vi "rs3 Set_calibration_table.vi"(8 "error in (no error)":errorcluster, 9 "calibration_Size":i32, 10 "PointerToNewCalibrationTable":u64, 11 "Device in":u64) -> (0 "error out":errorcluster, 1 "error":u64, 3 "Device out":u64)   [LabVIEW 2017, in "libRealSense3.lvlib"]
doc: "STARTS the streaming of a specific sensor, based on the input QUEUE."
uses:
  libRealSense3.lvlib
  realsense2.dll
panel:
  # "RS Set Calibration Table"
  # "(C) 2019 Intel Corp.,  AGJ"
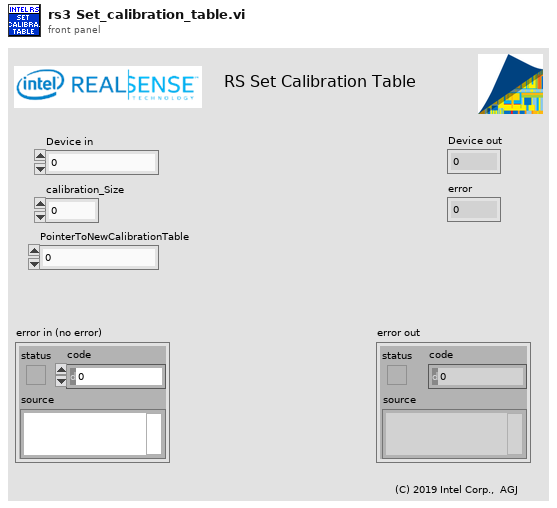
[diagram p1: front panel]
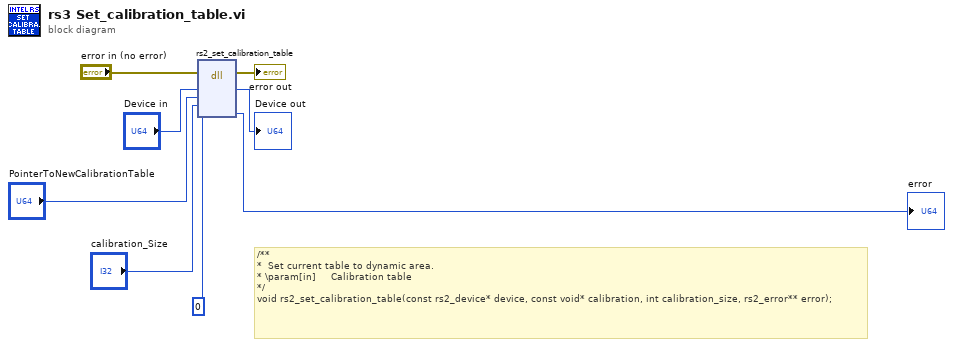
[diagram p0: block diagram]
diagram:
  # "/**\n*  Set current table to dynamic area.\n* \\param[in]     Calibration table\n*/\nvoid rs2_set_calibration_table(const rs2_device* device, const void* calibration, int calibration_size, rs2_error** error);"
  n1 = dll-call lib="C:/Users/agrunnet/Documents/libRealSense6/realsense2.dll" fn="rs2_set_calibration_table"(error in="error in (no error)", "device"="Device in", "CalibrationTable"="PointerToNewCalibrationTable", "calibration_Size"="calibration_Size", "error"=u64 0) -> (error out=→"error out":errorcluster, "device"=→"Device out":u64, "error"=→"error":u64)  [unwired: 5 in, 1 out]
